vi "SMTP Email SJIS.vi"(11 "text":string) -> (2 "isSJIS?":bool)   [LabVIEW 2012, in "NewNI_SMTPEmail.lvlib"]
uses:
  NewNI_SMTPEmail.lvlib
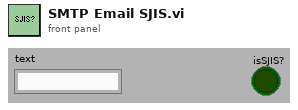
[diagram p1: front panel]
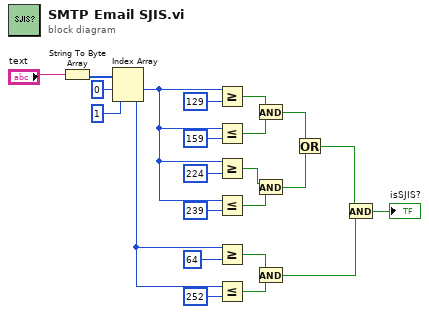
[diagram p0: block diagram]
diagram:
  n1 = String To Byte Array(string="text") -> (unsigned byte array=w23:u8[])
  n2 = Index Array(array=w23, index #1=0 ("index"), index #2=1 ("index")) -> (element #1=w13:u8, element #2=w6:u8)
  n3 = Greater Or Equal?(x=w13, y=u8 129) -> (x >= y?=w17:bool)
  n4 = Less Or Equal?(x=w13, y=u8 159) -> (x <= y?=w16:bool)
  n5 = Greater Or Equal?(x=w13, y=u8 224) -> (x >= y?=w12:bool)
  n6 = Less Or Equal?(x=w13, y=u8 239) -> (x <= y?=w11:bool)
  n7 = Greater Or Equal?(x=w6, y=u8 64) -> (x >= y?=w4:bool)
  n8 = Less Or Equal?(x=w6, y=u8 252) -> (x <= y?=w5:bool)
  n9 = And(x=w17, y=w16) -> (x .and. y?=w10:bool)
  n10 = And(x=w12, y=w11) -> (x .and. y?=w9:bool)
  n11 = And(x=w4, y=w5) -> (x .and. y?=w2:bool)
  n12 = Or(x=w10, y=w9) -> (x .or. y?=w3:bool)
  n13 = And(x=w3, y=w2) -> (x .and. y?=→"isSJIS?":bool)
